vi "Create All Message Queues.vi"(7 "max queue size (-1, unlimited)":i32=-1, 8 "error in (no error)":errorcluster) -> (0 "error out":errorcluster, 3 "Message Queues out":T1)   [LabVIEW 2016, in "Message Queue.lvlib"]
doc: "This VI creates and initializes all the message queues for your application. If your application requires more than one message queue, right-click the \"Message Queues\" constant above and select Open Type Def. Add the new Message Queue(s) to the type definition, then initialize them in this VI."
uses:
  Message Queue.lvlib
  All Message Queues.ctl
  Message Cluster.ctl
  Enqueue Message (Single).vi
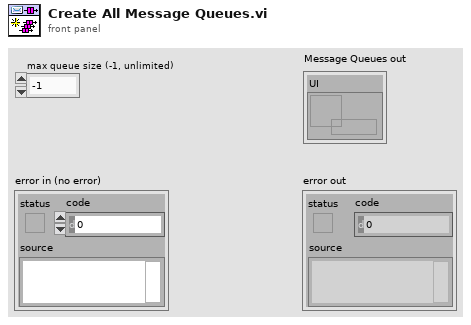
[diagram p1: front panel]
types:
  T1 = typedef "Message Queue.lvlib/All Message Queues.ctl" = cluster{"UI":refnum<queue>}
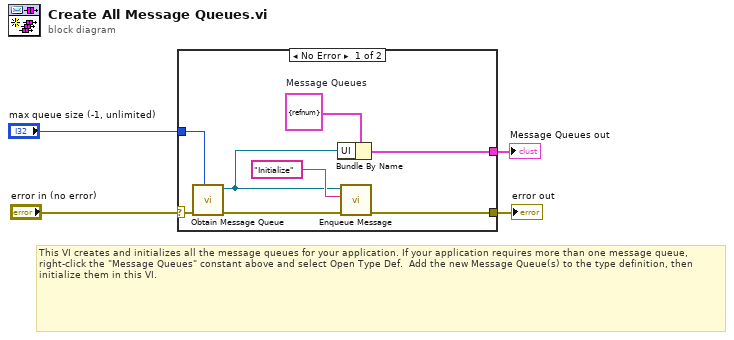
[diagram p0: block diagram]
diagram:
  # "This VI creates and initializes all the message queues for your application. If your application requires more than one message queue, right-click the \"Message Queues\" constant above and select Open Type Def.  Add the new Message Queue(s) to the type definition, then initialize them in this VI."
  n1 = case shown="No Error" "error in (no error)" {
    selector: "error in (no error)" -> [w9 w13]
    tunnel: [w12 w13] -> w4
    tunnel: [w10 _] -> w3
    tunnel: "max queue size (-1, unlimited)" -> [w5 _]
    frame No Error {
      w11 = T1 {"UI"=refnum}  # Message Queues
      n2 = call "Obtain Message Queue.vi"("max queue size (-1, unlimited)"=w5, "error in (no error)"=w9) -> ("error out"=w8:errorcluster, "Message Queue"=w6:refnum<queue>)  [unwired: 8 in]
      n3 = Bundle By Name(cluster=w11, "UI"=w6) -> (w10:T1)
      n4 = call-poly "Enqueue Message.vi"("error in (no error)"=w8, "Message"="Initialize", "Message Queue"=w6) -> ("error out"=w12:errorcluster)  [unwired: 7 in, 1 out]
    }
    frame Error {
    }
  }
  "Message Queues out" <- w3
  "error out" <- w4
